vi "Set Time.vi"(8 "error in (no error)":errorcluster, 9 "Command":enum16{"Set", "Get", "Pause", "Resume"}(ring), 10 "Target":dbl, 11 "Car Wash Controller in":refnum<class "Car Wash Controller.lvclass">) -> (0 "error out":errorcluster, 3 "Car Wash Controller out":refnum<class "Car Wash Controller.lvclass">)   [LabVIEW 2019]
uses:
  Sim Wash Display Console/Sim Wash Display Console Messages/Write Remaining timing Msg/Write Remaining timing Msg.lvclass
  Car Wash Controller.lvclass
  C:/Program Files (x86)/National Instruments/LabVIEW 2019/vi.lib/ActorFramework/Actor/Actor.lvclass
  <vilib>/ActorFramework/Message Enqueuer/Message Enqueuer.lvclass
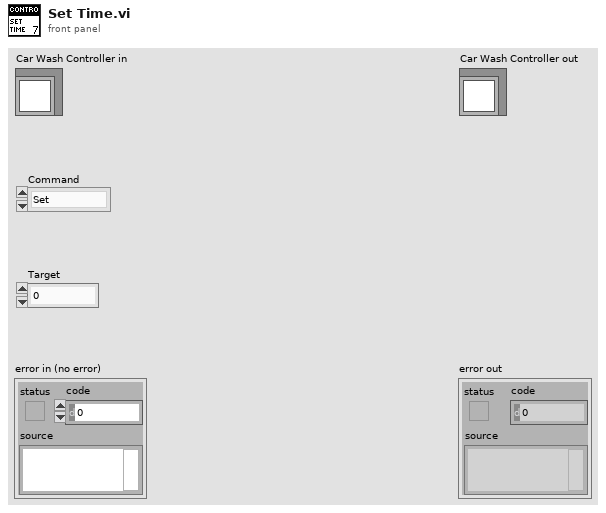
[diagram p1: front panel]
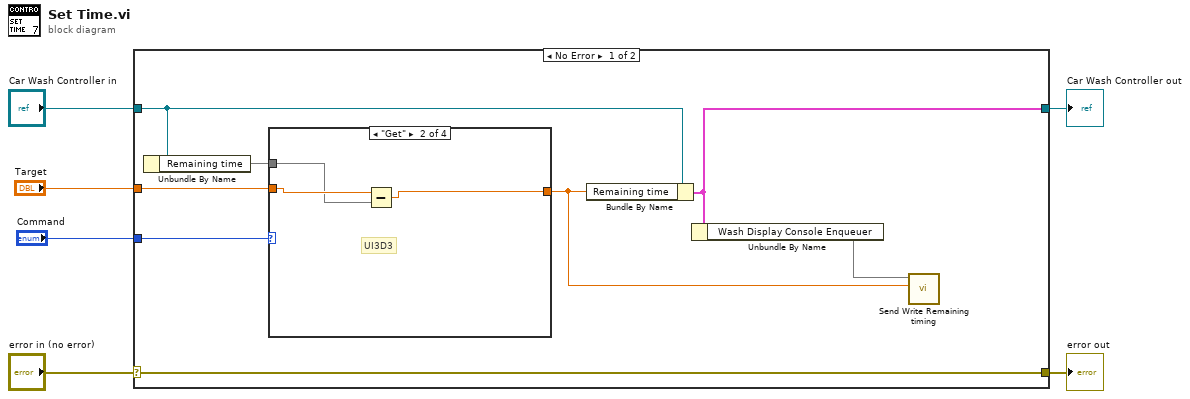
[diagram p0: block diagram]
diagram:
  n1 = case shown="No Error" "error in (no error)" {
    selector: "error in (no error)" -> [w14 w21]
    tunnel: [w14 w21] -> w5
    tunnel: [w9 w20] -> w3
    tunnel: "Car Wash Controller in" -> [w11 w20]
    tunnel: "Command" -> [w13 _]
    tunnel: "Target" -> [w12 _]
    frame No Error {
      n2 = Unbundle By Name(w11) -> ("Remaining time"=w10)
      n3 = case shown="\"Get\"" w13 {
        tunnel: w12 -> [w15 w18 _ _]
        tunnel: [w15 w16 _ w19] -> w7
        tunnel: w10 -> [_ w17 _ w19]
        frame "Set", Default {
        }
        frame "Get" {
          # "UI3D3"
          n4 = Subtract(x=w18, y=w17) -> (x-y=w16:dbl)
        }
        frame "Pause" {
        }
        frame "Resume" {
        }
      }
      n5 = Bundle By Name(cluster=w11, "Remaining time"=w7) -> (w9:cluster{})
      n6 = Unbundle By Name(w9) -> ("Wash Display Console Enqueuer"=w8)
      n7 = call "Send Write Remaining timing.vi"("Timing Remaining"=w7, "Message Enqueuer"=w8) -> ()  [unwired: 8 in, 2 out]
    }
    frame Error {
    }
  }
  "error out" <- w5
  "Car Wash Controller out" <- w3
